vi "StartDAQmxTasksControlVI.vi"(8 "entrée d'erreur (pas d'erreur)":errorcluster, 11 "Control en entrée":refnum<class "Control-Server.lvclass">) -> (0 "sortie d'erreur":errorcluster, 3 "Control en sortie":refnum<class "Control-Server.lvclass">)   [LabVIEW 2020, in "Control-Server.lvclass"]
uses:
  Control-Server.lvclass
  C:/dev/TRANCON/Classes/GeneralFunctionality/GeneralFunctionality.lvclass
  dependecies/ControlsVIs/Clusters-def/Message types.ctl
  Message/Message.lvclass/Message.ctl
  DAQmxTasks/DAQmxTaskContainer_General/DAQmxTaksContainer_General.lvclass
  Message/Message.lvclass
  GeneralFunctionality/GeneralFunctionality.lvclass
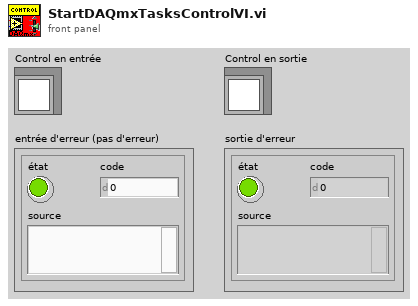
[diagram p1: front panel]
types:
  T1 = typedef "Message types.ctl" = string
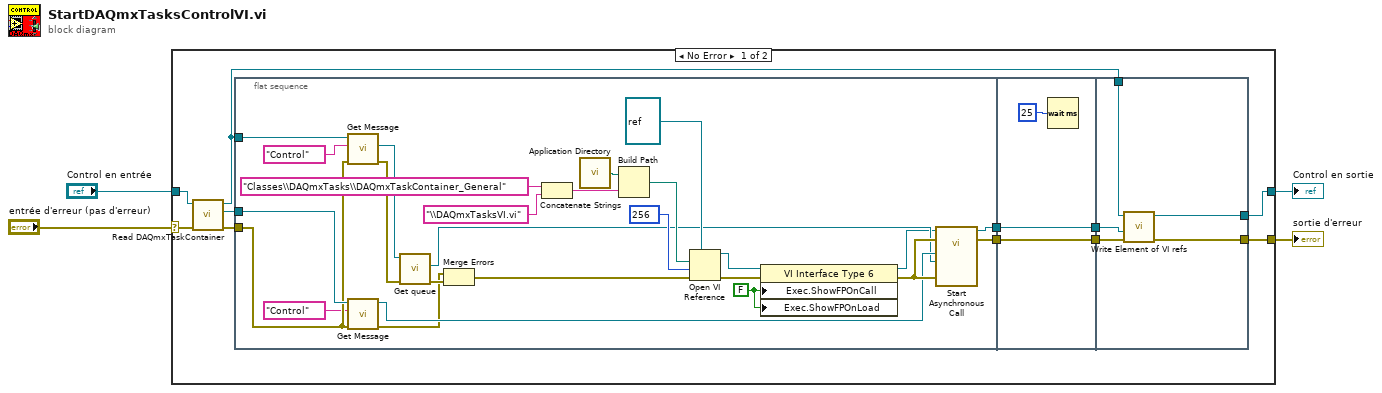
[diagram p0: block diagram]
diagram:
  n1 = case shown="No Error" "entrée d'erreur (pas d'erreur)" {
    selector: "entrée d'erreur (pas d'erreur)" -> [w13 w51]
    tunnel: [w15 w51] -> w4
    tunnel: "Control en entrée" -> [w14 w50]
    tunnel: [w10 w50] -> w2
    frame No Error {
      n2 = call-dynamic "Read DAQmxTaskContainer.vi"("error in (no error)"=w13, "Control in"=w14) -> ("error out"=w11:errorcluster, "DAQmxTaksContainer_General.lvclass"=w12:refnum<class "DAQmxTaksContainer_General.lvclass">, "Control out"=w9:refnum<class "Control-Server.lvclass">)  [unwired: 7 in]
      n3 = flat-sequence {
        tunnel: [w41] -> w8
        tunnel: [w30] -> w6
        tunnel: w11 -> [w27]
        tunnel: w9 -> [w29]
        tunnel: w12 -> [w28]
        tunnel: w8 -> [w44]
        tunnel: [w44] -> w7
        tunnel: w6 -> [w43]
        tunnel: [w43] -> w5
        tunnel: [w47] -> w15
        tunnel: w7 -> [w45]
        tunnel: [w49] -> w10
        tunnel: w5 -> [w48]
        tunnel: w9 -> [w46]
        frame #0 {
          w35 = FALSE ("Execution:Show Front Panel On Call")
          n4 = call "Get Message.vi"("error in (no error)"=w27, "Message type"=T1 "Control", "GeneralFunctionality en entrée"=w29) -> ("error out"=w21:errorcluster, "Message.lvclass"=w22:refnum<class "Message.lvclass">)  [unwired: 6 in, 1 out]
          n5 = call "Get Message.vi"("error in (no error)"=w27, "Message type"=T1 "Control", "GeneralFunctionality en entrée"=w28) -> ("error out"=w16:errorcluster, "GeneralFunctionality en sortie"=w25:refnum<class "DAQmxTaksContainer_General.lvclass">)  [unwired: 6 in, 1 out]
          n6 = call "Get queue.vi"("error in (no error)"=w21, "Message in"=w22) -> ("error out"=w20:errorcluster, "queue"=w18:refnum<queue>)  [unwired: 7 in, 1 out]
          n7 = Merge Errors(w16, w20) -> (w26:errorcluster)
          n8 = Concatenate Strings("Classes\\DAQmxTasks\\DAQmxTaskContainer_General" ("chaîne"), "\\DAQmxTasksVI.vi" ("chaîne")) -> (w33:string)
          n9 = call <vilib>:"Application Directory.vi"() -> ("Application Directory"=w39:path)
          n10 = Build Path(base path=w39, name or relative path=w33) -> (appended path=w40:path)
          n11 = Open VI Reference(type specifier VI Refnum (for type only)=refnum<vi> refnum ("spécificateur de type du refnum de VI (pour type seulement)"), vi path=w40, options=256, error in (no error)=w26) -> (vi reference=w19:refnum<vi>, error out=w36:errorcluster)  [unwired: 2 in]
          n12 = property class="VI Interface Type 6"(reference=w19, error in=w36, "Exec.ShowFPOnCall"=w35, "Exec.ShowFPOnLoad"=w35) -> (reference out=w17:refnum<vi>, error out=w34:errorcluster)
          n13 = call-by-ref "Start Asynchronous Call"(reference=w17, error in=w34, 8:"error in (no error)"=w34, "ControlQueue"=w18, "DAQmxTaksContainer_General.lvclass"=w25) -> (reference out=w30:refnum<vi>, error out=w41:errorcluster)  [unwired: 9 in]
        }
        frame #1 {
          n14 = Wait (ms)(milliseconds to wait=u32 25) -> ()  [unwired: 1 out]
        }
        frame #2 {
          n15 = call "Write Element of VI refs.vi"("error in (no error)"=w45, "vi reference"=w48, "Control in"=w46) -> ("error out"=w47:errorcluster, "Control out"=w49:refnum<class "Control-Server.lvclass">)  [unwired: 7 in]
        }
      }
    }
    frame Error {
    }
  }
  "sortie d'erreur" <- w4
  "Control en sortie" <- w2
